vi "FTW-TestStep-Base_StartTime.vi"(0 "FTW-TestStep-Base In":refnum<class "FTW-TestStep-Base.lvclass">, 11 "error in (no error)":errorcluster) -> (4 "FTW-TestStep-Base Out":refnum<class "FTW-TestStep-Base.lvclass">, 15 "error out":errorcluster)   [LabVIEW 2015, in "FTW-TestStep-Base.lvclass"]
uses:
  FTW-TestStep-Base.lvclass
  FTW-TestStep-Base.lvclass/FTW-TestStep-Base.ctl
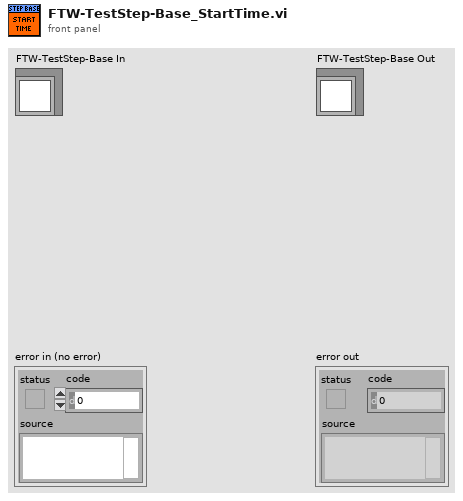
[diagram p1: front panel]
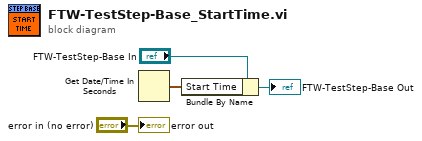
[diagram p0: block diagram]
diagram:
  n1 = Get Date/Time In Seconds() -> (seconds since 1Jan1904=w1:timestamp)
  n2 = Bundle By Name(cluster="FTW-TestStep-Base In", "Start Time"=w1) -> (→"FTW-TestStep-Base Out":refnum<class "FTW-TestStep-Base.lvclass">)
  "error out" <- "error in (no error)"
